vi "Change.vi"(8 "Error In":errorcluster, 11 "總辨識結果":string[](array[string])) -> (0 "Error Out":errorcluster, 3 "輸出顏色-位置":T1(array[cluster]))   [LabVIEW 2019]
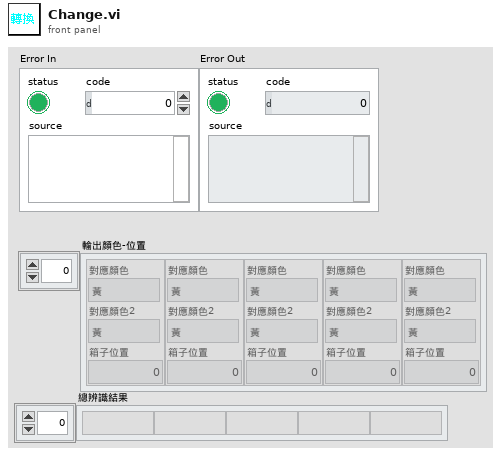
[diagram p1: front panel]
types:
  T1 = cluster{"對應顏色":enum16{"黃", "紅", "綠", "藍", "黑", "無"}, "對應顏色2":enum16{"黃", "紅", "綠", "藍", "黑", "無"}, "箱子位置":i32}[]
  T2 = cluster{"對應顏色":enum16{"黃", "紅", "綠", "藍", "黑", "無"}, "對應顏色2":enum16{"黃", "紅", "綠", "藍", "黑", "無"}, "箱子位置":i32}
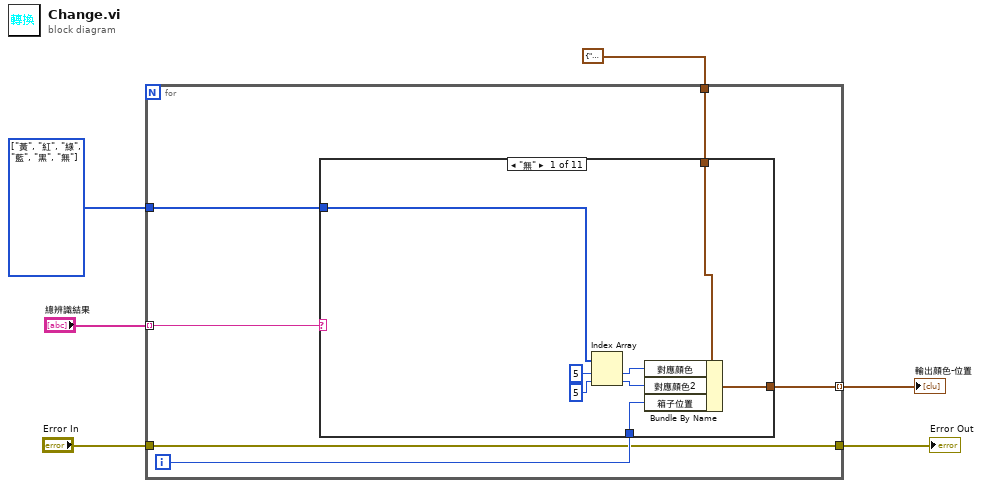
[diagram p0: block diagram]
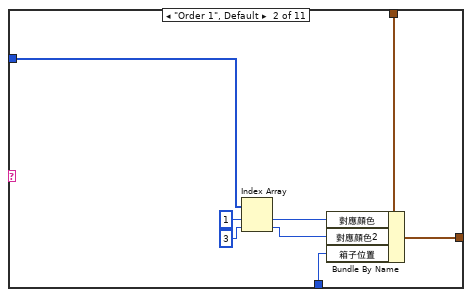
[diagram p2: hidden frame]
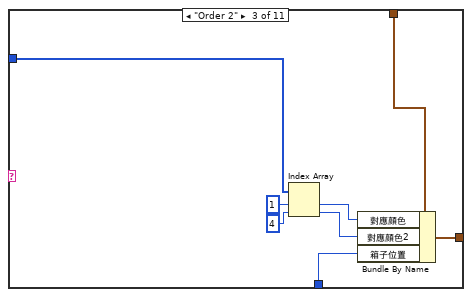
[diagram p3: hidden frame]
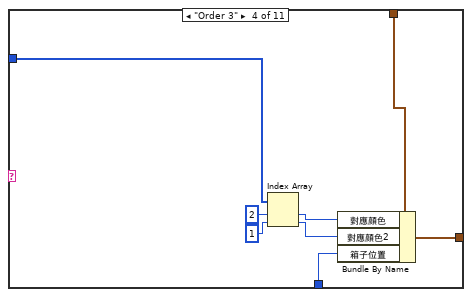
[diagram p4: hidden frame]
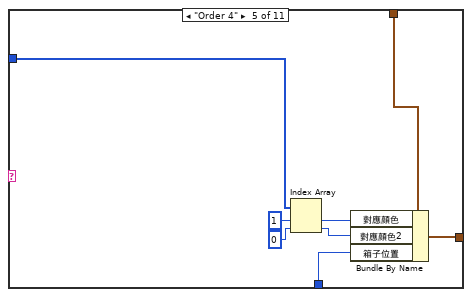
[diagram p5: hidden frame]
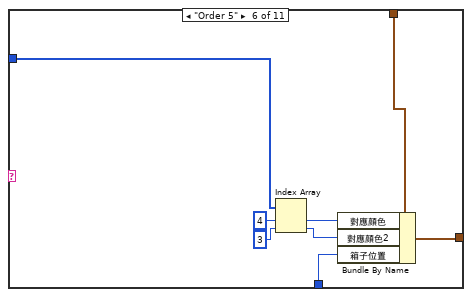
[diagram p6: hidden frame]
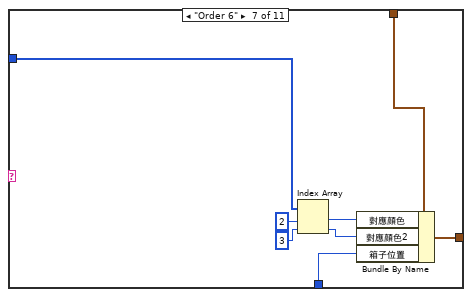
[diagram p7: hidden frame]
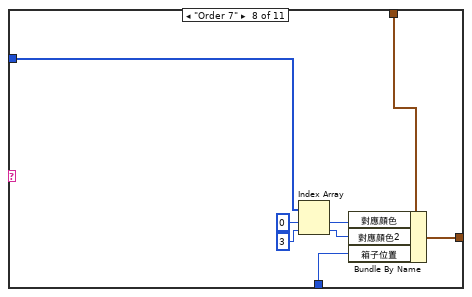
[diagram p8: hidden frame]
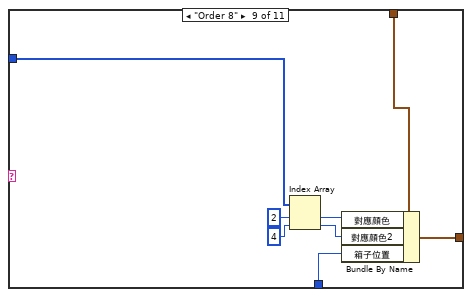
[diagram p9: hidden frame]
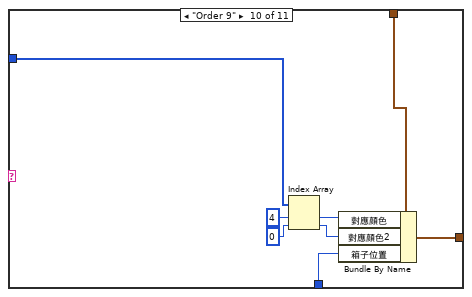
[diagram p10: hidden frame]
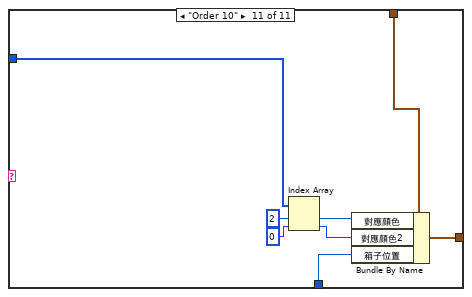
[diagram p11: hidden frame]
diagram:
  w1 = enum16{"黃", "紅", "綠", "藍", "黑", "無"}[] [enum."黃", enum."紅", enum."綠", enum."藍", enum."黑", enum."無"] items=["黃", "紅", "綠", "藍", "黑", "無"]
  n1 = for {
    tunnel: [w11] -> w6 mode=indexing
    tunnel: "總辨識結果" -> [w9] mode=indexing
    tunnel: [w10] -> w5
    tunnel: "Error In" -> [w10]
    tunnel: T2 {"對應顏色"=enum."黃", "對應顏色2"=enum."黃", "箱子位置"=0} ("input cluster") -> [w8]
    tunnel: w1 -> [w7]
    i -> [w12]
    n2 = case shown="\"無\"" w9 {
      tunnel: w12 -> [w19 w28 w35 w44 w51 w59 w67 w75 w83 w91 w99]
      tunnel: [w20 w27 w36 w43 w52 w60 w68 w76 w84 w92 w100] -> w11
      tunnel: w8 -> [w18 w26 w34 w42 w50 w58 w66 w74 w82 w90 w98]
      tunnel: w7 -> [w13 w21 w29 w37 w45 w53 w61 w69 w77 w85 w93]
      frame "無" {
        n3 = Index Array(array=w13, index #1=5 ("index"), index #2=5 ("index")) -> (element #1=w15:enum16{"黃", "紅", "綠", "藍", "黑", "無"}, element #2=w14:enum16{"黃", "紅", "綠", "藍", "黑", "無"})
        n4 = Bundle By Name(cluster=w18, "對應顏色"=w15, "對應顏色2"=w14, "箱子位置"=w19) -> (w20:T2)
      }
      frame "Order 1", Default {
        n5 = Index Array(array=w21, index #1=1 ("index"), index #2=3 ("index")) -> (element #1=w25:enum16{"黃", "紅", "綠", "藍", "黑", "無"}, element #2=w24:enum16{"黃", "紅", "綠", "藍", "黑", "無"})
        n6 = Bundle By Name(cluster=w26, "對應顏色"=w25, "對應顏色2"=w24, "箱子位置"=w28) -> (w27:T2)
      }
      frame "Order 2" {
        n7 = Index Array(array=w29, index #1=1 ("index"), index #2=4 ("index")) -> (element #1=w31:enum16{"黃", "紅", "綠", "藍", "黑", "無"}, element #2=w30:enum16{"黃", "紅", "綠", "藍", "黑", "無"})
        n8 = Bundle By Name(cluster=w34, "對應顏色"=w31, "對應顏色2"=w30, "箱子位置"=w35) -> (w36:T2)
      }
      frame "Order 3" {
        n9 = Index Array(array=w37, index #1=2 ("index"), index #2=1 ("index")) -> (element #1=w39:enum16{"黃", "紅", "綠", "藍", "黑", "無"}, element #2=w38:enum16{"黃", "紅", "綠", "藍", "黑", "無"})
        n10 = Bundle By Name(cluster=w42, "對應顏色"=w39, "對應顏色2"=w38, "箱子位置"=w44) -> (w43:T2)
      }
      frame "Order 4" {
        n11 = Index Array(array=w45, index #1=1 ("index"), index #2=0 ("index")) -> (element #1=w47:enum16{"黃", "紅", "綠", "藍", "黑", "無"}, element #2=w46:enum16{"黃", "紅", "綠", "藍", "黑", "無"})
        n12 = Bundle By Name(cluster=w50, "對應顏色"=w47, "對應顏色2"=w46, "箱子位置"=w51) -> (w52:T2)
      }
      frame "Order 5" {
        n13 = Index Array(array=w53, index #1=4 ("index"), index #2=3 ("index")) -> (element #1=w55:enum16{"黃", "紅", "綠", "藍", "黑", "無"}, element #2=w54:enum16{"黃", "紅", "綠", "藍", "黑", "無"})
        n14 = Bundle By Name(cluster=w58, "對應顏色"=w55, "對應顏色2"=w54, "箱子位置"=w59) -> (w60:T2)
      }
      frame "Order 6" {
        n15 = Index Array(array=w61, index #1=2 ("index"), index #2=3 ("index")) -> (element #1=w63:enum16{"黃", "紅", "綠", "藍", "黑", "無"}, element #2=w62:enum16{"黃", "紅", "綠", "藍", "黑", "無"})
        n16 = Bundle By Name(cluster=w66, "對應顏色"=w63, "對應顏色2"=w62, "箱子位置"=w67) -> (w68:T2)
      }
      frame "Order 7" {
        n17 = Index Array(array=w69, index #1=0 ("index"), index #2=3 ("index")) -> (element #1=w71:enum16{"黃", "紅", "綠", "藍", "黑", "無"}, element #2=w70:enum16{"黃", "紅", "綠", "藍", "黑", "無"})
        n18 = Bundle By Name(cluster=w74, "對應顏色"=w71, "對應顏色2"=w70, "箱子位置"=w75) -> (w76:T2)
      }
      frame "Order 8" {
        n19 = Index Array(array=w77, index #1=2 ("index"), index #2=4 ("index")) -> (element #1=w79:enum16{"黃", "紅", "綠", "藍", "黑", "無"}, element #2=w78:enum16{"黃", "紅", "綠", "藍", "黑", "無"})
        n20 = Bundle By Name(cluster=w82, "對應顏色"=w79, "對應顏色2"=w78, "箱子位置"=w83) -> (w84:T2)
      }
      frame "Order 9" {
        n21 = Index Array(array=w85, index #1=4 ("index"), index #2=0 ("index")) -> (element #1=w87:enum16{"黃", "紅", "綠", "藍", "黑", "無"}, element #2=w86:enum16{"黃", "紅", "綠", "藍", "黑", "無"})
        n22 = Bundle By Name(cluster=w90, "對應顏色"=w87, "對應顏色2"=w86, "箱子位置"=w91) -> (w92:T2)
      }
      frame "Order 10" {
        n23 = Index Array(array=w93, index #1=2 ("index"), index #2=0 ("index")) -> (element #1=w95:enum16{"黃", "紅", "綠", "藍", "黑", "無"}, element #2=w94:enum16{"黃", "紅", "綠", "藍", "黑", "無"})
        n24 = Bundle By Name(cluster=w98, "對應顏色"=w95, "對應顏色2"=w94, "箱子位置"=w99) -> (w100:T2)
      }
    }
  }
  "Error Out" <- w5
  "輸出顏色-位置" <- w6
